vi "ChangeTimer.vi"(2 "TravelTime (ms)":u32=2000, 3 "CheckValue":dbl) -> (1 "Finished?":bool)   [LabVIEW 2017, in "ArgosLib.lvlib"]
uses:
  ArgosLib.lvlib
panel:
  # "Timer to indicate when a specified amount of time has elapsed after a change in CheckValue\nUseful to do rough completion estimation for pneumatic cylinders"
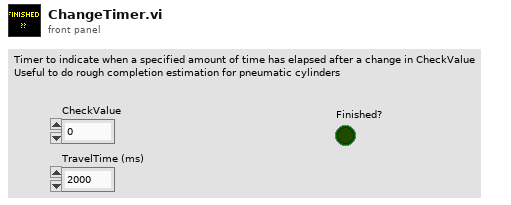
[diagram p1: front panel]
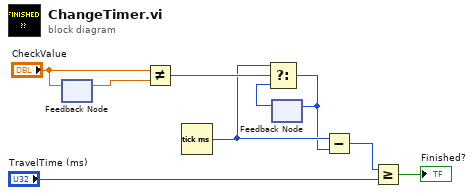
[diagram p0: block diagram]
diagram:
  n1 = feedback-in #1("CheckValue") -> ()
  n2 = feedback #1() -> (w6:dbl)  [unwired: 1 in]
  n3 = Not Equal?(x="CheckValue", y=w6) -> (x != y?=w5:bool)
  n4 = Tick Count (ms)() -> (millisecond timer value=w3:u32)
  n5 = feedback #2() -> (w1:u32)  [unwired: 1 in]
  n6 = Select(t=w3, s=w5, f=w1) -> (s? t:f=w2:u32)
  n7 = feedback-in #2(w2) -> ()
  n8 = Subtract(x=w3, y=w2) -> (x-y=w4:u32)
  n9 = Greater Or Equal?(x=w4, y="TravelTime (ms)") -> (x >= y?=→"Finished?":bool)
